vi "Temperatura y motor ino .vi"() -> ()   [LabVIEW 2013]
uses:
  <vilib>/Instr/_visa.llb/VISA Configure Serial Port (Instr).vi
panel:
  out "Waveform Chart":i32(graph)
  out "Estado del motor":bool
  out "Termómetro °C":dbl(slide) scale=0.0..90.0
  out "Temperatura °C":string
  in  "VISA resource name":refnum<visa-resource-name>
  in  "Controlar motor":bool
  # "SENSOR DE TEMPERATURA CON INTERFAZ GRÁFICA"
  # "Acondicionamiento de señales eléctricas"
  # "Allan Daniel Macedo Méndez"
  # "COMUNICACIÓN SERIAL"
  # "MOTOR"
  # "INDICADORES DE TEMPERATURA"
  # "Setpoint: 50 °C"
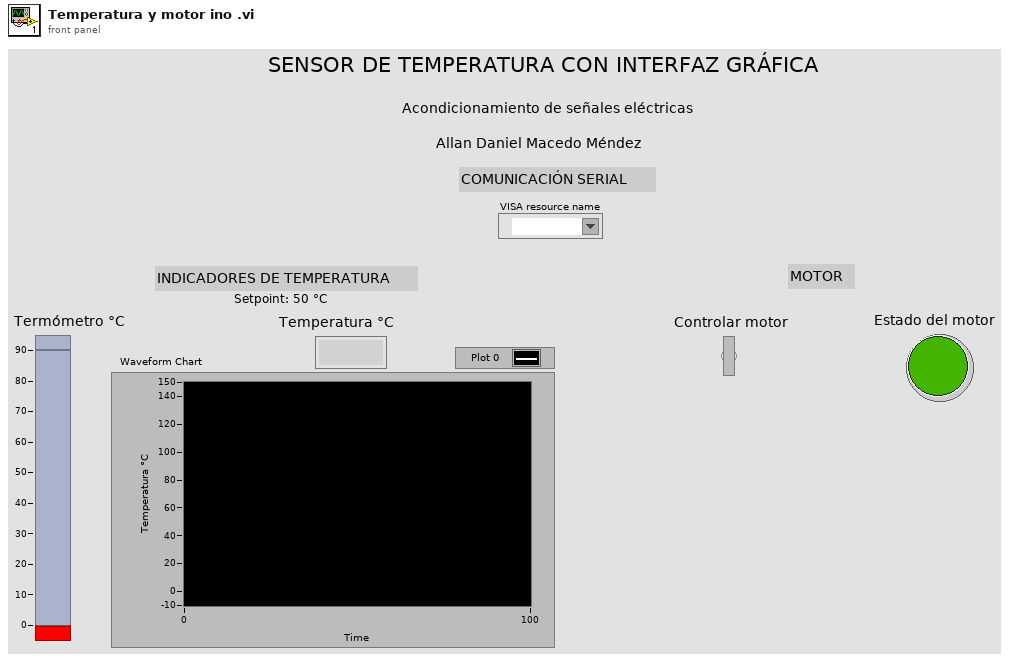
[diagram p1: front panel]
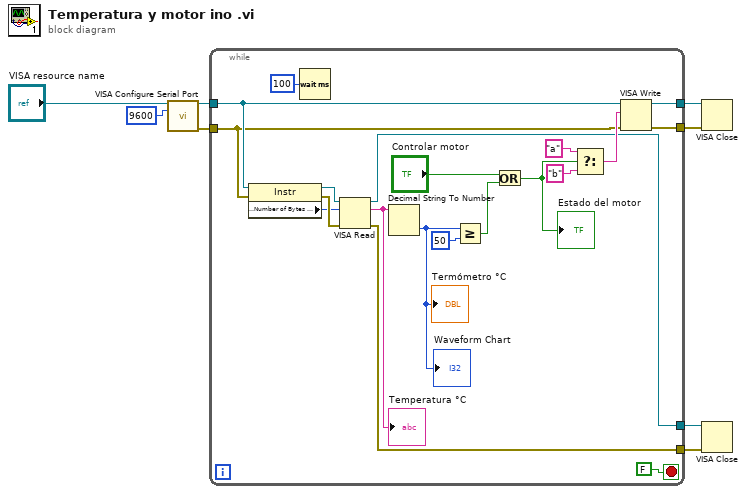
[diagram p0: block diagram]
diagram:
  n1 = call-poly "VISA Configure Serial Port"("VISA resource name"="VISA resource name", "baud rate (9600)"=9600) -> ("VISA resource name out"=w6:refnum<visa-resource-name>, "error out"=w5:errorcluster)  [unwired: 12 in]
  n2 = while {
    tunnel: w6 -> [w23]
    tunnel: w5 -> [w22]
    tunnel: [w25] -> w3
    tunnel: [w24] -> w4
    tunnel: [w18] -> w1
    tunnel: [w17] -> w2
    stop <- FALSE stop-if-true
    n3 = property class="Instr"(reference=w23, error in=w22) -> (reference out=w21:refnum<visa-resource-name>, error out=w20:errorcluster, "Serial Settings:Number of Bytes at Serial Port"=w19:u32)
    n4 = Wait (ms)(milliseconds to wait=100) -> ()  [unwired: 1 out]
    n5 = VISA Read(VISA resource name=w21, byte count=w19, error in (no error)=w20) -> (VISA resource name out=w18:refnum<visa-resource-name>, read buffer=w15:string, error out=w17:errorcluster)  [unwired: 1 out]
    "Temperatura °C" <- w15
    n6 = Decimal String To Number(string=w15) -> (number=w9:i32)  [unwired: 2 in, 1 out]
    "Termómetro °C" <- w9
    "Waveform Chart" <- w9
    n7 = Greater Or Equal?(x=w9, y=50) -> (x >= y?=w11:bool)
    n8 = Or(x="Controlar motor", y=w11) -> (x .or. y?=w10:bool)
    "Estado del motor" <- w10
    n9 = Select(t="a", s=w10, f="b") -> (s? t:f=w26:string)
    n10 = VISA Write(VISA resource name=w23, write buffer=w26, error in (no error)=w22) -> (VISA resource name out=w25:refnum<visa-resource-name>, error out=w24:errorcluster)  [unwired: 1 out]
  }
  n11 = VISA Close(VISA resource name=w3, error in (no error)=w4) -> ()  [unwired: 1 out]
  n12 = VISA Close(VISA resource name=w1, error in (no error)=w2) -> ()  [unwired: 1 out]
